vi "DRWM_DSF.vi"(5 "棒限值":dbl[](array[numeric]), 7 "DRWM开":bool, 8 "动态棒位":dbl, 9 "DSF因子":cluster{"x":dbl, "y":dbl}[][](array[cluster]), 10 "上下段通量选择":u16[](array[numeric]), 11 "反应性in":dbl[](array[numeric])) -> (3 "反应性out":dbl[](array[numeric]))   [LabVIEW 2020]
uses:
  <vilib>/Analysis/baseanly.llb/Mean (DBL).vi
  <vilib>/Analysis/NI_AALBase.lvlib
panel:
  out "下段":dbl caption="下段降棒前正反应性" format="%0.2f"
  out "上段":dbl caption="上段降棒前正反应性" format="%0.2f"
  out "反应性积累":dbl[][](array[numeric])
  out "棒位积累":dbl[](array[numeric])
  in  "棒位到底":bool
  in  "落棒前正反应性":dbl[][](array[numeric])
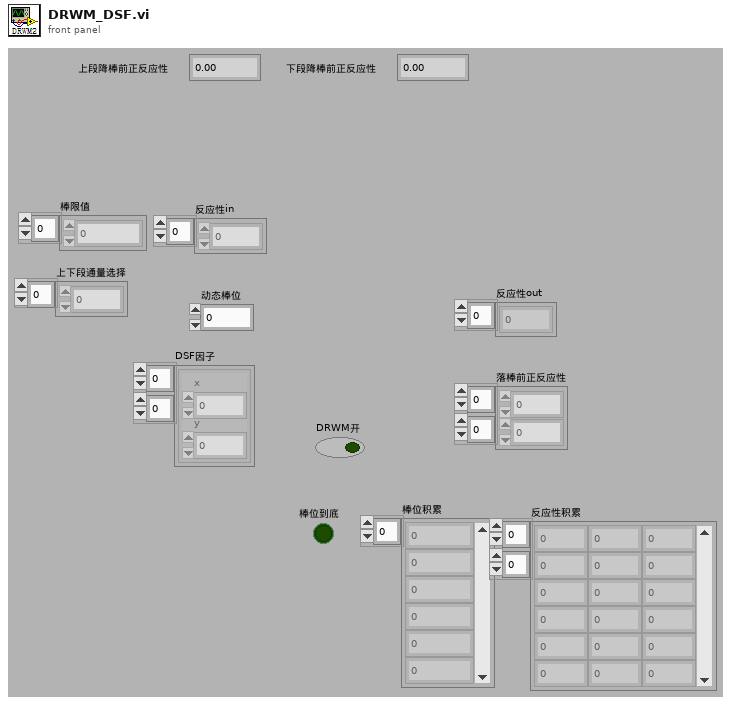
[diagram p1: front panel]
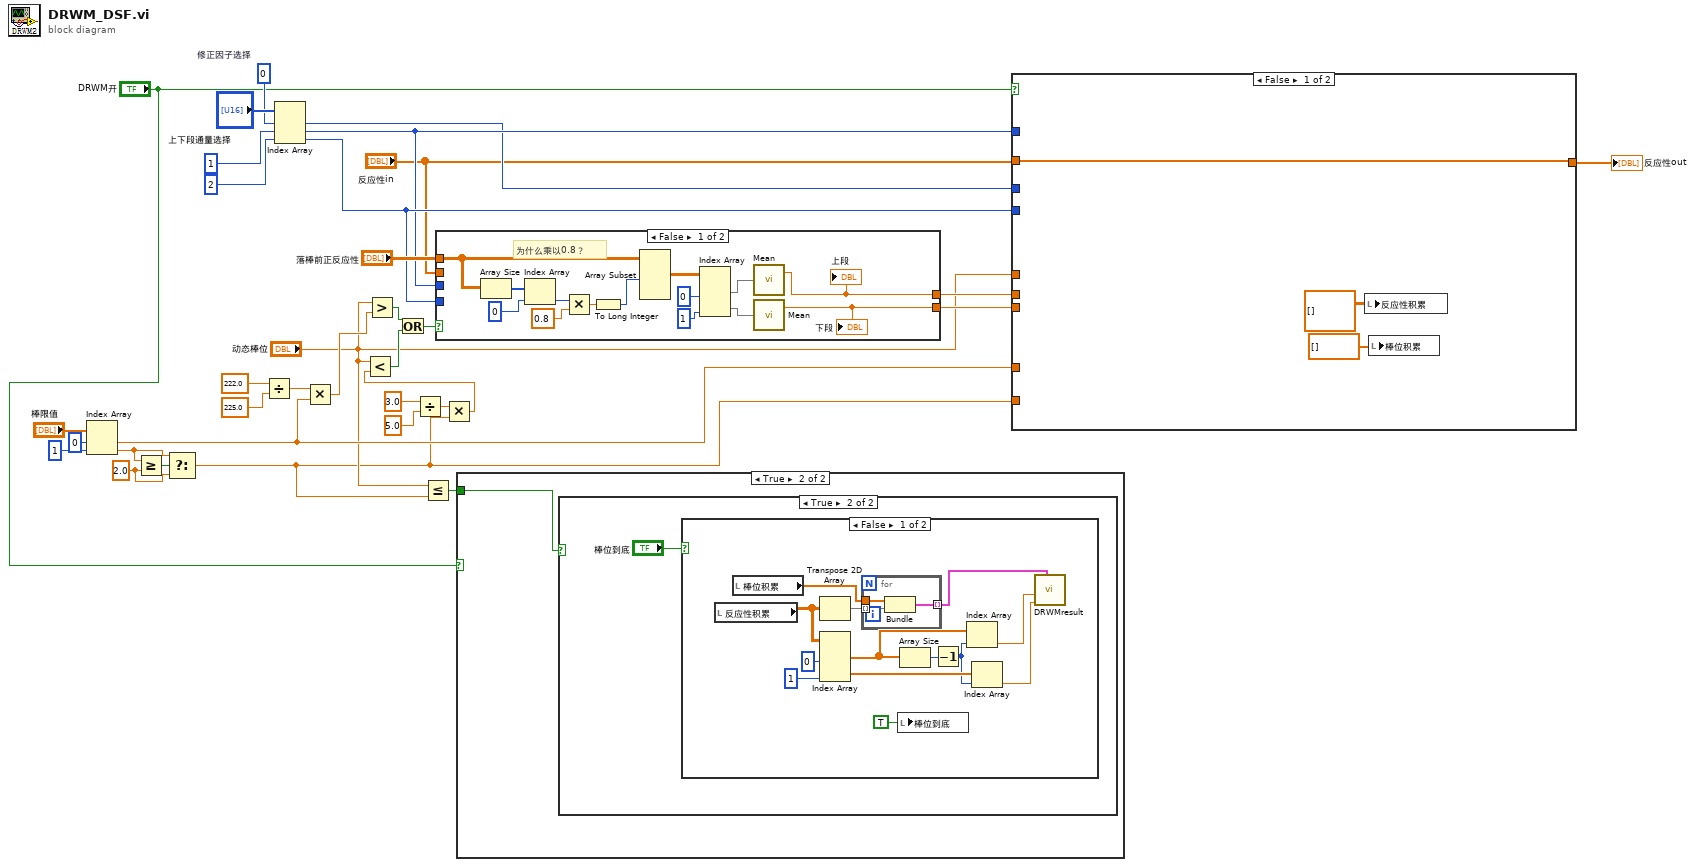
[diagram p0: block diagram]
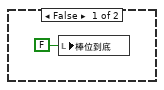
[diagram p2: hidden frame]
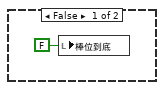
[diagram p3: hidden frame]
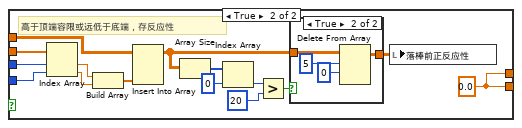
[diagram p5: hidden frame]
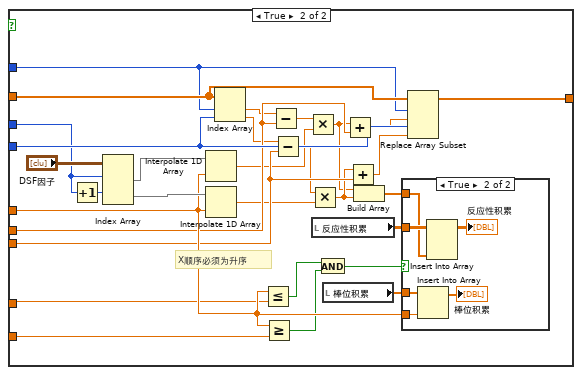
[diagram p7: hidden frame]
diagram:
  w12 = 2.0 ("y")
  w15 = 0  # 修正因子选择
  n1 = Index Array(array="棒限值", index #1=0 ("索引"), index #2=1 ("索引")) -> (element #1=w25:dbl, element #2=w13:dbl)
  n2 = Greater Or Equal?(x=w13, y=w12) -> (x >= y?=w14:bool)
  n3 = Select(t=w13, s=w14, f=w12) -> (s? t:f=w3:dbl)
  n4 = Divide(x=222.0, y=225.0) -> (x/y=w24:dbl)
  n5 = Index Array(array="上下段通量选择", index #1=w15, index #2=1 ("索引"), index #3=2 ("索引")) -> (element #1=w9:u16, element #2=w10:u16, element #3=w11:u16)
  n6 = Multiply(x=w24, y=w25) -> (x*y=w21:dbl)
  n7 = Greater?(x="动态棒位", y=w21) -> (0:w31:bool)
  n8 = Divide(x=3.0, y=5.0) -> (x/y=w20:dbl)
  n9 = Less Or Equal?(x="动态棒位", y=w3) -> (x <= y?=w1:bool)
  n10 = Multiply(x=w20, y=w3) -> (x*y=w17:dbl)
  n11 = Less?(x="动态棒位", y=w17) -> (x < y?=w30:bool)
  n12 = Or(x=w31, y=w30) -> (x .or. y?=w29:bool)
  n13 = case shown="False" w29 {
    tunnel: "反应性in" -> [_ w63]
    tunnel: w10 -> [_ w62]
    tunnel: w11 -> [_ w61]
    tunnel: "落棒前正反应性" -> [w48 w50]
    tunnel: [w36 w49] -> w33
    tunnel: [w35 w49] -> w32
    frame False {
      # "为什么乘以0.8？"
      n14 = Array Size(array=w48) -> (size(s)=w47:i32[])
      n15 = Index Array(array=w47, index=0 ("索引")) -> (element=w45:i32)
      n16 = Multiply(x=w45, y=0.8 ("元素")) -> (x*y=w43:dbl)
      n17 = To Long Integer(number=w43) -> (32bit integer=w42:i32)
      n18 = Array Subset(array=w48, length (row)=w42) -> (w41:dbl[][])  [unwired: 3 in]
      n19 = Index Array(array=w41, index (col) #1=0 ("禁用的索引 (列)"), index (col) #2=1 ("索引 (列)")) -> (element #1=w38:dbl[], element #2=w37:dbl[])  [unwired: 2 in]
      n20 = call-poly <vilib>:"Mean.vi"("X"=w38) -> ("mean"=w36:dbl)  [unwired: 1 out]
      "上段" <- w36
      n21 = call-poly <vilib>:"Mean.vi"("X"=w37) -> ("mean"=w35:dbl)  [unwired: 1 out]
      "下段" <- w35
    }
    frame True {
      w49 = 0.0 ("mean")
      # "高于顶端容限或远低于底端，存反应性"
      n22 = Index Array(array=w63, index #1=w62, index #2=w61) -> (element #1=w60:dbl, element #2=w59:dbl)
      n23 = Build Array(w60, w59) -> (w58:dbl[])
      n24 = Insert Into Array(array=w50, new element=w58) -> (w57:dbl[][])  [unwired: 2 in]
      n25 = Array Size(array=w57) -> (size(s)=w55:i32[])
      n26 = Index Array(array=w55, index=0 ("索引")) -> (element=w53:i32)
      n27 = Greater?(x=w53, y=20) -> (0:w51:bool)
      n28 = case shown="True" w51 {
        tunnel: w57 -> [w64 w68]
        tunnel: [w64 w67] -> w56
        frame False {
        }
        frame True {
          n29 = Delete From Array(array=w68, length=5 ("长度"), index (row)=0 ("索引 (行)")) -> (array with subset deleted=w67:dbl[][])  [unwired: 1 in, 1 out]
        }
      }
      n30 = local write "落棒前正反应性"(w56) -> ()
    }
  }
  n31 = case shown="True" "DRWM开" {
    tunnel: w1 -> [_ w70]
    frame False {
      n32 = local write "棒位到底"(FALSE ("棒位到底")) -> ()
    }
    frame True {
      n33 = case shown="True" w70 {
        frame False {
          n34 = local write "棒位到底"(FALSE ("棒位到底")) -> ()
        }
        frame True {
          n35 = case shown="False" "棒位到底" {
            frame False {
              n36 = local read "反应性积累"() -> (w78:dbl[][])
              n37 = local read "棒位积累"() -> (w76:dbl[])
              n38 = Transpose 2D Array(2D array=w78) -> (transposed array=w77:dbl[][])
              n39 = Index Array(array=w78, index (col) #1=0 ("禁用的索引 (列)"), index (col) #2=1 ("索引 (列)")) -> (element #1=w80:dbl[], element #2=w83:dbl[])  [unwired: 2 in]
              n40 = for {
                tunnel: w76 -> [w86]
                tunnel: w77 -> [w87] mode=indexing
                tunnel: [w88] -> w79 mode=indexing
                n41 = Bundle "Bundle"("棒位积累"=w86, w87) -> (w88:cluster{"棒位积累":dbl[], dbl[]})  [unwired: 1 in]
              }
              n42 = local write "棒位到底"(TRUE ("棒位到底")) -> ()
              n43 = Array Size(array=w80) -> (size(s)=w81:i32)
              n44 = Decrement(x=w81) -> (x-1=w82:i32)
              n45 = Index Array(array=w80, index=w82) -> (element=w84:dbl)
              n46 = Index Array(array=w83, index=w82) -> (element=w85:dbl)
              n47 = call "DRWMresult.vi"("价值曲线"=w79, "下段总价值"=w85, "上段总价值"=w84) -> ()  [unwired: 9 in]
            }
            frame True {
            }
          }
        }
      }
    }
  }
  n48 = case shown="False" "DRWM开" {
    tunnel: [w91 w121] -> w4
    tunnel: "反应性in" -> [w91 w117]
    tunnel: "动态棒位" -> [_ w116]
    tunnel: w11 -> [_ w115]
    tunnel: w10 -> [_ w114]
    tunnel: w33 -> [_ w113]
    tunnel: w32 -> [_ w112]
    tunnel: w25 -> [_ w111]
    tunnel: w3 -> [_ w110]
    tunnel: w9 -> [_ w108]
    frame False {
      n49 = local write "反应性积累"(dbl[][] [] ("反应性积累")) -> ()
      n50 = local write "棒位积累"(dbl[] [] ("棒位积累")) -> ()
    }
    frame True {
      # "X顺序必须为升序"
      n51 = Increment(x=w108) -> (x+1=w109:u16)
      n52 = Index Array(array="DSF因子", index (row) #1=w108, index (row) #2=w109) -> (element #1=w119:cluster{"x":dbl, "y":dbl}[], element #2=w118:cluster{"x":dbl, "y":dbl}[])  [unwired: 2 in]
      n53 = Interpolate 1D Array(1:w116, 2:w119) -> (0:w107:dbl)
      n54 = Interpolate 1D Array(1:w116, 2:w118) -> (0:w106:dbl)
      n55 = Index Array(array=w117, index #1=w114, index #2=w115) -> (element #1=w105:dbl, element #2=w104:dbl)
      n56 = Less Or Equal?(x=w116, y=w111) -> (x <= y?=w94:bool)
      n57 = Greater Or Equal?(x=w116, y=w110) -> (x >= y?=w95:bool)
      n58 = Subtract(x=w105, y=w113) -> (x-y=w102:dbl)
      n59 = Subtract(x=w104, y=w112) -> (x-y=w103:dbl)
      n60 = Multiply(x=w102, y=w107) -> (x*y=w92:dbl)
      n61 = Multiply(x=w103, y=w106) -> (x*y=w93:dbl)
      n62 = local read "反应性积累"() -> (w98:dbl[][])
      n63 = And(x=w94, y=w95) -> (x .and. y?=w96:bool)
      n64 = local read "棒位积累"() -> (w99:dbl[])
      n65 = Add(x=w92, y=w113) -> (x+y=w101:dbl)
      n66 = Add(x=w93, y=w112) -> (x+y=w100:dbl)
      n67 = Build Array(w92, w93) -> (w97:dbl[])
      n68 = case shown="True" w96 {
        tunnel: w99 -> [_ w127]
        tunnel: w116 -> [_ w125]
        tunnel: w98 -> [_ w123]
        tunnel: w97 -> [_ w122]
        frame False {
        }
        frame True {
          n69 = Insert Into Array(array=w127, new element=w125) -> (→"棒位积累":dbl[])  [unwired: 1 in]
          n70 = Insert Into Array(array=w123, new element=w122) -> (→"反应性积累":dbl[][])  [unwired: 2 in]
        }
      }
      n71 = Replace Array Subset(array=w117, new element #1=w101, index #1=w114, new element #2=w100, index #2=w115) -> (w121:dbl[])
    }
  }
  "反应性out" <- w4
